vi "ICR_Update_Controls.vi"(7 "Command":T1, 8 "error in (no error)":errorcluster caption="entrée d'erreur (pas d'erreur)", 11 "QMH ICR Cluster":T2) -> (0 "error out":errorcluster caption="sortie d'erreur", 3 "QMH ICR Cluster":T2)   [LabVIEW 2024]
doc: "This VI enables or disables controls according to QMH command."
uses:
  controls/QMH_ICR_Cluster.ctl
  controls/HARDWARE_Resources.ctl
  controls/PROCESSING_Inputs.ctl
  controls/LOOPS_Inputs.ctl
  controls/OPO_Inputs.ctl
  controls/QMH_ICR_Command.ctl
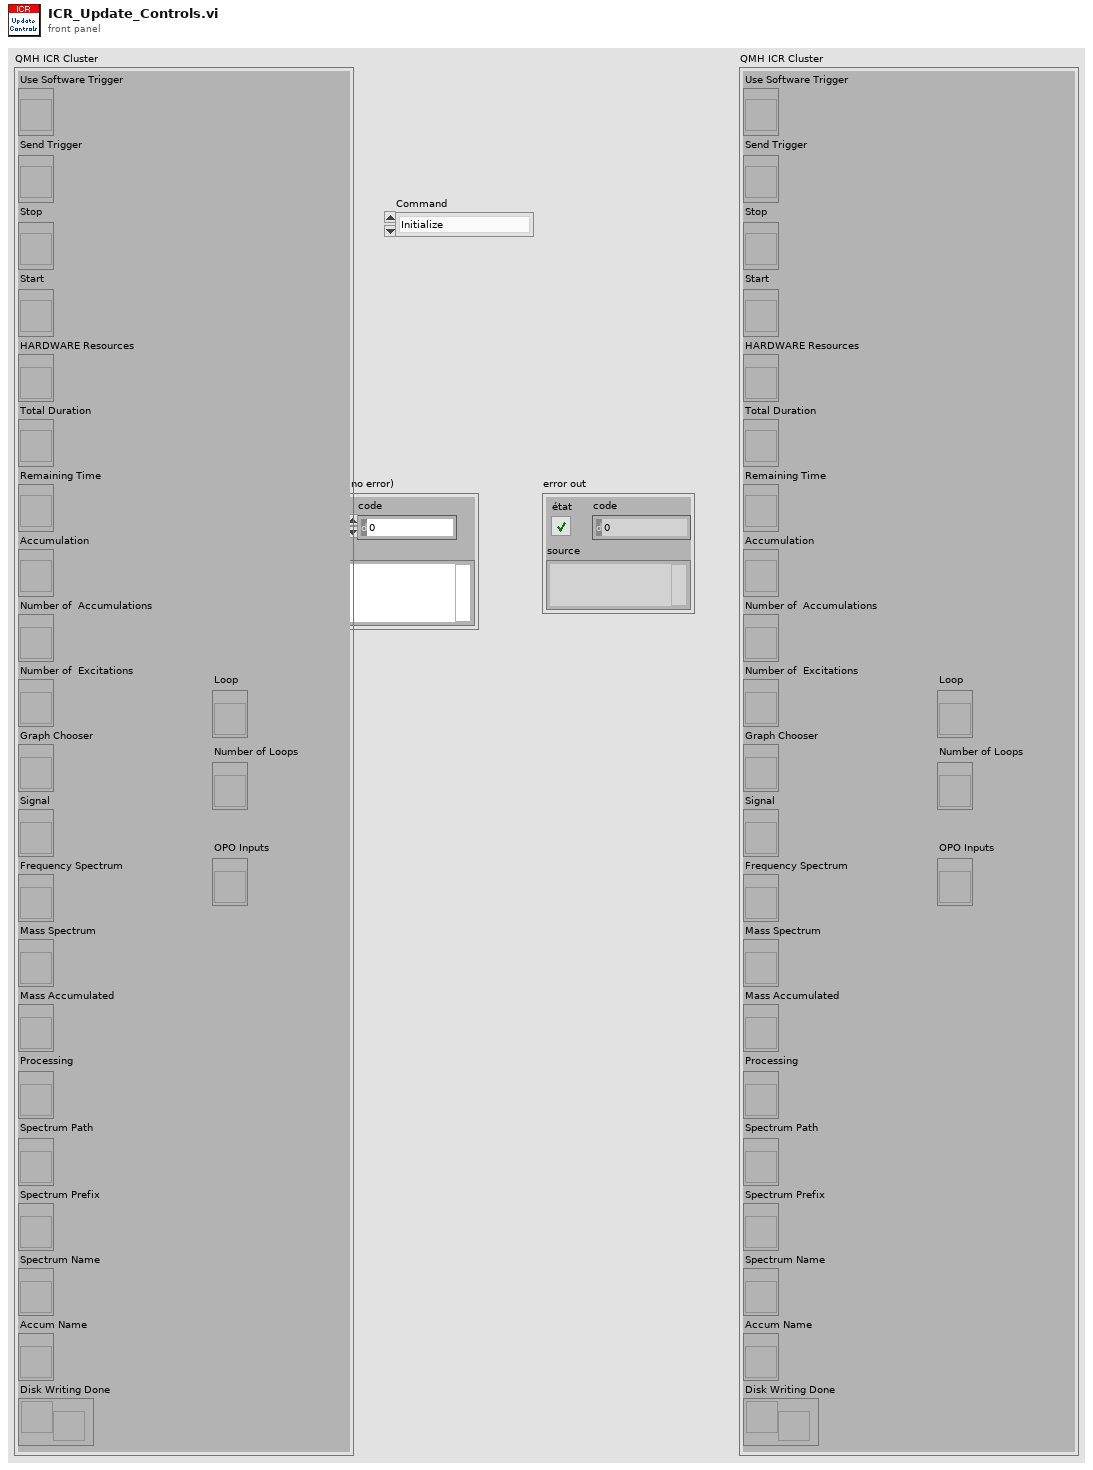
[diagram p1: front panel]
types:
  T1 = typedef "QMH_ICR_Command.ctl" = enum16{"Initialize", "Sequence Loop Setup", "Sequence Setup", "ICR Start", "ICR Stop", "Hardware Setup", "Next Sequence Loop", "Next Accumulation", "Waiting for Trigger", "Sequence Started", "Sequence Finished", "Sequence Loop Done", "Writing Data", "Hardware Reset", "Exit"}
  T2 = typedef "QMH_ICR_Cluster.ctl" = cluster{"Use Software Trigger":refnum<vi>, "Send Trigger":refnum<vi>, "Stop":refnum<vi>, "Start":refnum<vi>, "HARDWARE Resources":refnum<vi>, "Total Duration":refnum<vi>, "Remaining Time":refnum<vi>, "Accumulation":refnum<vi>, "Number of  Accumulations":refnum<vi>, "Number of  Excitations":refnum<vi>, "Graph Chooser":refnum<vi>, "Signal":refnum<vi>, "Frequency Spectrum":refnum<vi>, "Mass Spectrum":refnum<vi>, "Mass Accumulated":refnum<vi>, "Processing":refnum<vi>, "Spectrum Path":refnum<vi>, "Spectrum Prefix":refnum<vi>, "Spectrum Name":refnum<vi>, "Accum Name":refnum<vi>, "Disk Writing Done":refnum<notifier>, "Loop":refnum<vi>, "Number of Loops":refnum<vi>, "OPO Inputs":refnum<vi>}
  T3 = enum32{"Signal", "Frequency Spectrum", "Mass Spectrum", "Mass Accumulated"}
  T4 = enum8{"Enabled", "Disabled", "Disabled and Grayed Out"}
  T5 = typedef "PROCESSING_Inputs.ctl" = cluster{"Reference Mass":dbl, "Cyclotron Freq":dbl, "Magnetron Freq":dbl}
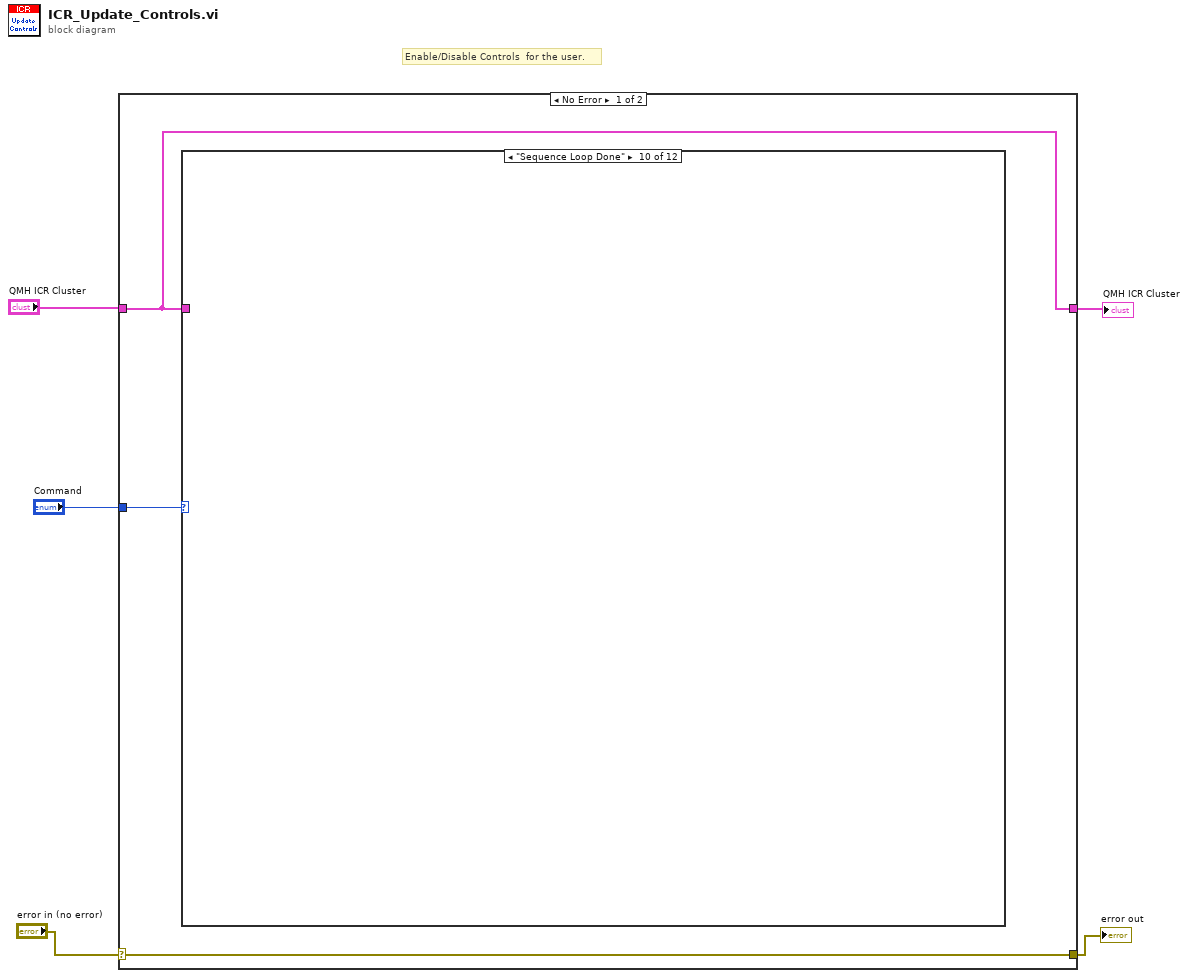
[diagram p0: block diagram]
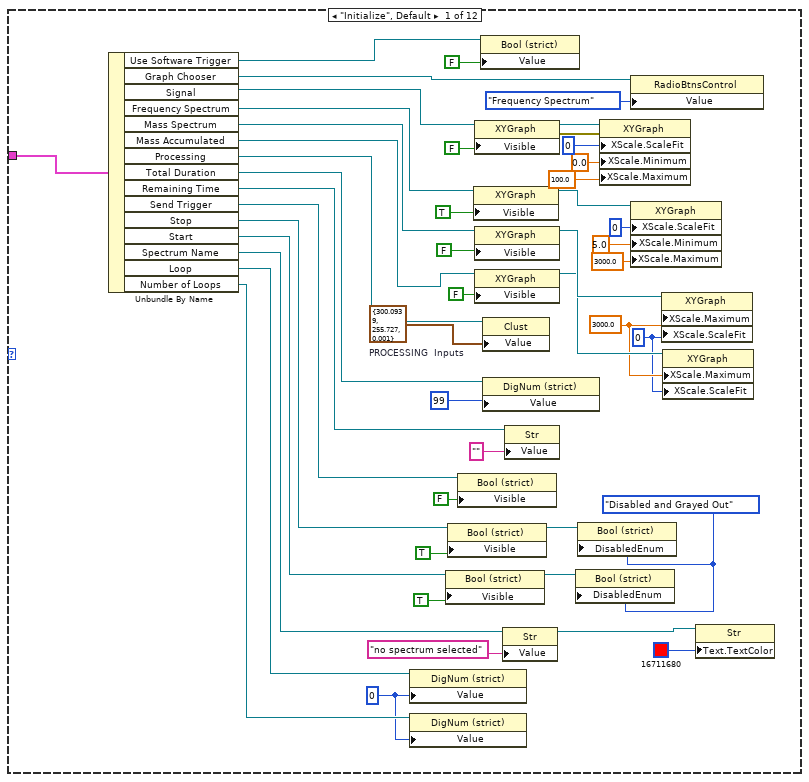
[diagram p2: hidden frame]
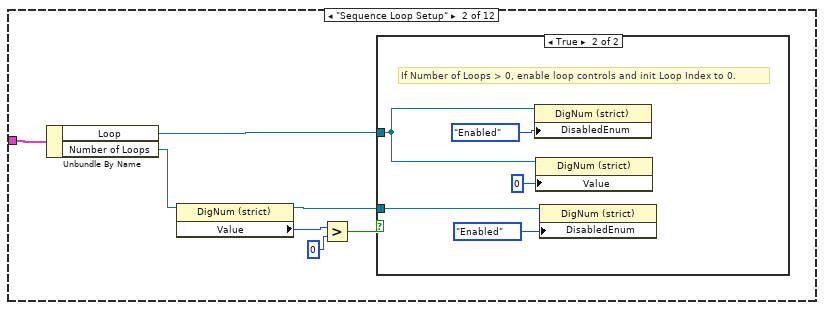
[diagram p3: hidden frame]
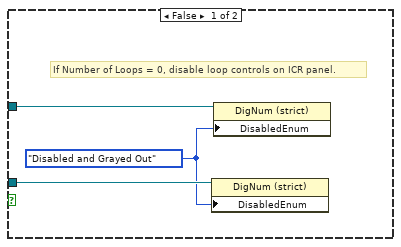
[diagram p4: hidden frame]
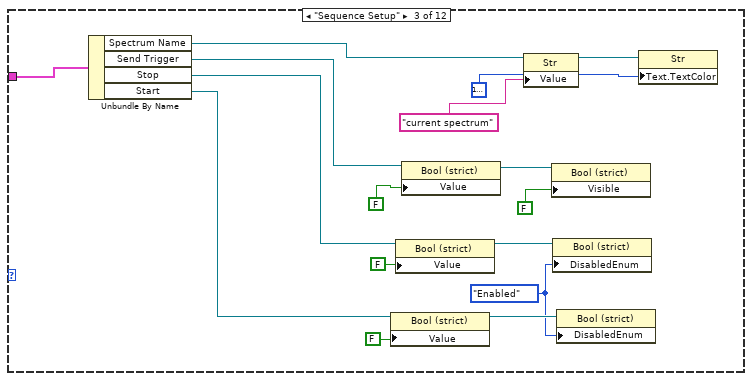
[diagram p5: hidden frame]
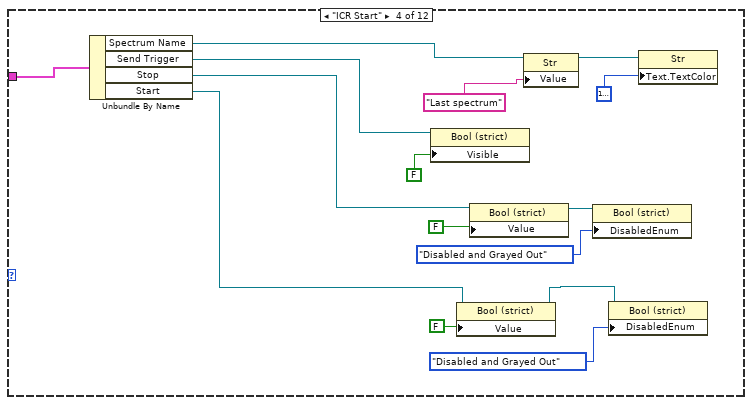
[diagram p6: hidden frame]
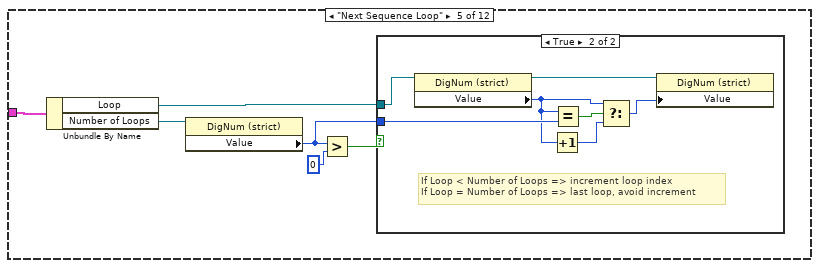
[diagram p7: hidden frame]
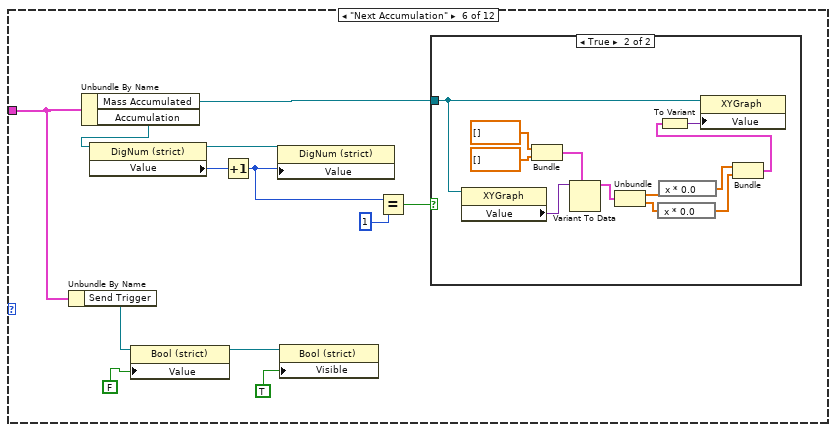
[diagram p9: hidden frame]
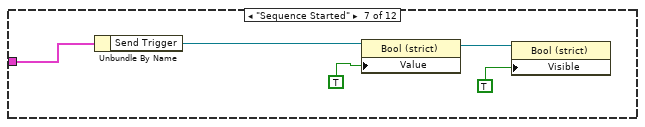
[diagram p11: hidden frame]
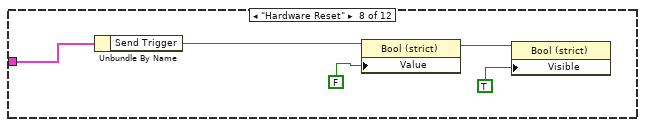
[diagram p12: hidden frame]
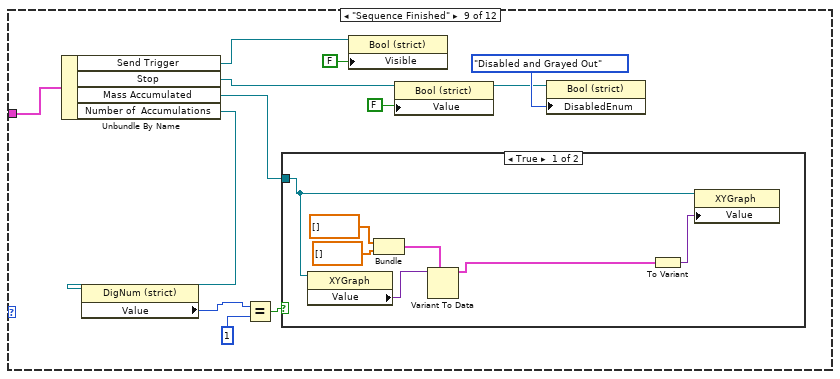
[diagram p13: hidden frame]
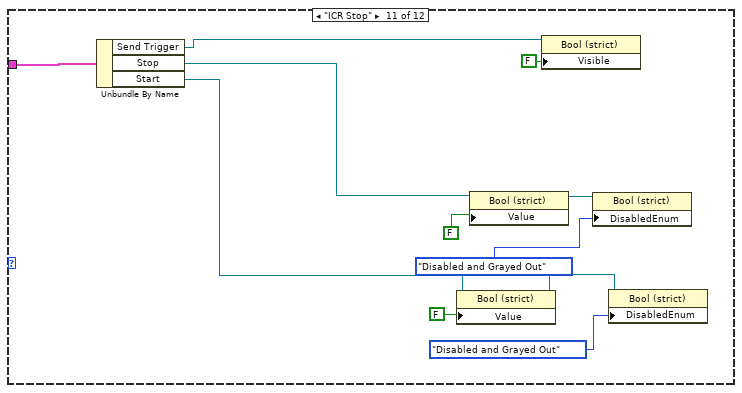
[diagram p15: hidden frame]
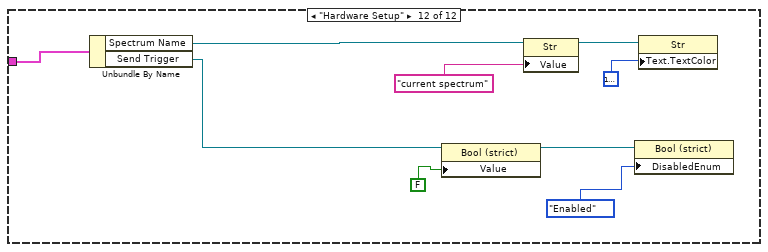
[diagram p16: hidden frame]
diagram:
  # "Enable/Disable Controls  for the user."
  n1 = case shown="No Error" "error in (no error)" {
    selector: "error in (no error)" -> [w8 w190]
    tunnel: "QMH ICR Cluster" -> [w7 w189]
    tunnel: [w8 w190] -> w2
    tunnel: [w7 w189] -> w5
    tunnel: "Command" -> [w6 _]
    frame No Error {
      n2 = case shown="\"Sequence Loop Done\"" w6 {
        tunnel: w7 -> [w32 w63 w87 w102 w108 w117 w144 w149 w161 _ w179 w188]
        frame "Initialize", Default {
          w9 = i16 0 ("Value")
          w16 = u8 0 ("Échelle des X.Ajuster l'échelle")
          w17 = 3000.0 ("Échelle des X.Gamme:Minimum")
          w25 = T4."Disabled and Grayed Out" ("Désactivé")
          w35 = T5 {"Reference Mass"=300.0939, "Cyclotron Freq"=255.727, "Magnetron Freq"=0.001}  # PROCESSING  Inputs
          n3 = Unbundle By Name(w32) -> ("Use Software Trigger"=w48:refnum<vi>, "Graph Chooser"=w49:refnum<vi>, "Signal"=w50:refnum<vi>, "Frequency Spectrum"=w51:refnum<vi>, "Mass Spectrum"=w52:refnum<vi>, "Mass Accumulated"=w36:refnum<vi>, "Processing"=w42:refnum<vi>, "Total Duration"=w46:refnum<vi>, "Remaining Time"=w44:refnum<vi>, "Send Trigger"=w29:refnum<vi>, "Stop"=w39:refnum<vi>, "Start"=w26:refnum<vi>, "Spectrum Name"=w30:refnum<vi>, "Loop"=w11:refnum<vi>, "Number of Loops"=w10:refnum<vi>)
          n4 = property class="DigNum (strict)"(reference=w11, "Value"=w9) -> ()  [unwired: 1 in, 2 out]
          n5 = property class="DigNum (strict)"(reference=w10, "Value"=w9) -> ()  [unwired: 1 in, 2 out]
          n6 = property class="Bool (strict)"(reference=w26, "Visible"=TRUE) -> (reference out=w28:refnum<vi>)  [unwired: 1 in, 1 out]
          n7 = property class="Bool (strict)"(reference=w39, "Visible"=TRUE) -> (reference out=w34:refnum<vi>)  [unwired: 1 in, 1 out]
          n8 = property class="Bool (strict)"(reference=w29, "Visible"=FALSE) -> ()  [unwired: 1 in, 2 out]
          n9 = property class="XYGraph"(reference=w51, "Visible"=TRUE) -> (reference out=w21:refnum<vi>)  [unwired: 1 in, 1 out]
          n10 = property class="XYGraph"(reference=w50, "Visible"=FALSE) -> (reference out=w24:refnum<vi>, error out=w23:errorcluster)  [unwired: 1 in]
          n11 = property class="XYGraph"(reference=w52, "Visible"=FALSE) -> (reference out=w19:refnum<vi>)  [unwired: 1 in, 1 out]
          n12 = property class="XYGraph"(reference=w36, "Visible"=FALSE) -> (reference out=w18:refnum<vi>)  [unwired: 1 in, 1 out]
          n13 = property class="Bool (strict)"(reference=w48, "Value"=FALSE ("Valeur")) -> ()  [unwired: 1 in, 2 out]
          n14 = property class="Clust"(reference=w42, "Value"=w35) -> ()  [unwired: 1 in, 2 out]
          n15 = property class="DigNum (strict)"(reference=w46, "Value"=99) -> ()  [unwired: 1 in, 2 out]
          n16 = property class="Str"(reference=w30, "Value"="no spectrum selected" ("Valeur")) -> (reference out=w40:refnum<vi>)  [unwired: 1 in, 1 out]
          n17 = property class="Str"(reference=w44, "Value"="" ("Valeur")) -> ()  [unwired: 1 in, 2 out]
          n18 = property class="Bool (strict)"(reference=w28, "DisabledEnum"=w25) -> ()  [unwired: 1 in, 2 out]
          n19 = property class="Bool (strict)"(reference=w34, "DisabledEnum"=w25) -> ()  [unwired: 1 in, 2 out]
          n20 = property class="XYGraph"(reference=w24, error in=w23, "XScale.ScaleFit"=u8 0 ("Échelle des X.Ajuster l'échelle"), "XScale.Minimum"=0.0 ("Échelle des X.Gamme:Minimum"), "XScale.Maximum"=100.0 ("Échelle des X.Gamme:Maximum")) -> ()  [unwired: 2 out]
          n21 = property class="RadioBtnsControl"(reference=w49, "Value"=T3."Frequency Spectrum" ("Graph Chooser")) -> ()  [unwired: 1 in, 2 out]
          n22 = property class="XYGraph"(reference=w21, "XScale.ScaleFit"=u8 0 ("Échelle des X.Ajuster l'échelle"), "XScale.Minimum"=5.0 ("Échelle des X.Gamme:Minimum"), "XScale.Maximum"=3000.0 ("Échelle des X.Gamme:Maximum")) -> ()  [unwired: 1 in, 2 out]
          n23 = property class="XYGraph"(reference=w19, "XScale.Maximum"=w17, "XScale.ScaleFit"=w16) -> ()  [unwired: 1 in, 2 out]
          n24 = property class="XYGraph"(reference=w18, "XScale.Maximum"=w17, "XScale.ScaleFit"=w16) -> ()  [unwired: 1 in, 2 out]
          n25 = property on="Nœud de propriété" class="Str"(reference=w40, "Text.TextColor"=u32 16711680) -> ()  [unwired: 1 in, 2 out]
        }
        frame "Sequence Loop Setup" {
          n26 = Unbundle By Name(w63) -> ("Loop"=w60:refnum<vi>, "Number of Loops"=w58:refnum<vi>)
          n27 = property class="DigNum (strict)"(reference=w58) -> (reference out=w57:refnum<vi>, "Value"=w59:i16)  [unwired: 1 in, 1 out]
          n28 = Greater?(x=w59, y=i16 0) -> (0:w62:bool)
          n29 = case shown="True" w62 {
            tunnel: w60 -> [w66 w69]
            tunnel: w57 -> [w65 w71]
            frame False {
              w64 = T4."Disabled and Grayed Out" ("Disabled")
              # "If Number of Loops = 0, disable loop controls on ICR panel."
              n30 = property class="DigNum (strict)"(reference=w65, "DisabledEnum"=w64) -> ()  [unwired: 1 in, 2 out]
              n31 = property class="DigNum (strict)"(reference=w66, "DisabledEnum"=w64) -> ()  [unwired: 1 in, 2 out]
            }
            frame True {
              # "If Number of Loops > 0, enable loop controls and init Loop Index to 0."
              n32 = property class="DigNum (strict)"(reference=w69, "DisabledEnum"=T4."Enabled" ("Disabled")) -> ()  [unwired: 1 in, 2 out]
              n33 = property class="DigNum (strict)"(reference=w69, "Value"=i16 0) -> ()  [unwired: 1 in, 2 out]
              n34 = property class="DigNum (strict)"(reference=w71, "DisabledEnum"=T4."Enabled" ("Disabled")) -> ()  [unwired: 1 in, 2 out]
            }
          }
        }
        frame "Sequence Setup" {
          w72 = T4."Enabled" ("Désactivé")
          n35 = Unbundle By Name(w87) -> ("Spectrum Name"=w85:refnum<vi>, "Send Trigger"=w82:refnum<vi>, "Stop"=w77:refnum<vi>, "Start"=w73:refnum<vi>)
          n36 = property class="Bool (strict)"(reference=w73, "Value"=FALSE ("Valeur")) -> (reference out=w75:refnum<vi>)  [unwired: 1 in, 1 out]
          n37 = property class="Bool (strict)"(reference=w77, "Value"=FALSE ("Valeur")) -> (reference out=w78:refnum<vi>)  [unwired: 1 in, 1 out]
          n38 = property class="Bool (strict)"(reference=w82, "Value"=FALSE ("Valeur")) -> (reference out=w81:refnum<vi>)  [unwired: 1 in, 1 out]
          n39 = property class="Str"(reference=w85, "Value"="current spectrum" ("Valeur")) -> (reference out=w83:refnum<vi>)  [unwired: 1 in, 1 out]
          n40 = property class="Bool (strict)"(reference=w81, "Visible"=FALSE) -> ()  [unwired: 1 in, 2 out]
          n41 = property class="Bool (strict)"(reference=w78, "DisabledEnum"=w72) -> ()  [unwired: 1 in, 2 out]
          n42 = property class="Bool (strict)"(reference=w75, "DisabledEnum"=w72) -> ()  [unwired: 1 in, 2 out]
          n43 = property on="Nœud de propriété" class="Str"(reference=w83, "Text.TextColor"=u32 16777222) -> ()  [unwired: 1 in, 2 out]
        }
        frame "ICR Start" {
          n44 = Unbundle By Name(w102) -> ("Spectrum Name"=w101:refnum<vi>, "Send Trigger"=w89:refnum<vi>, "Stop"=w97:refnum<vi>, "Start"=w94:refnum<vi>)
          n45 = property class="Bool (strict)"(reference=w89, "Visible"=FALSE) -> ()  [unwired: 1 in, 2 out]
          n46 = property class="Bool (strict)"(reference=w94, "Value"=FALSE ("Valeur")) -> (reference out=w95:refnum<vi>)  [unwired: 1 in, 1 out]
          n47 = property class="Bool (strict)"(reference=w97, "Value"=FALSE ("Valeur")) -> (reference out=w98:refnum<vi>)  [unwired: 1 in, 1 out]
          n48 = property class="Str"(reference=w101, "Value"="Last spectrum" ("Valeur")) -> (reference out=w99:refnum<vi>)  [unwired: 1 in, 1 out]
          n49 = property class="Bool (strict)"(reference=w98, "DisabledEnum"=T4."Disabled and Grayed Out" ("Désactivé")) -> ()  [unwired: 1 in, 2 out]
          n50 = property class="Bool (strict)"(reference=w95, "DisabledEnum"=T4."Disabled and Grayed Out" ("Désactivé")) -> ()  [unwired: 1 in, 2 out]
          n51 = property on="Nœud de propriété" class="Str"(reference=w99, "Text.TextColor"=u32 16777222) -> ()  [unwired: 1 in, 2 out]
        }
        frame "Next Sequence Loop" {
          n52 = Unbundle By Name(w108) -> ("Loop"=w104:refnum<vi>, "Number of Loops"=w106:refnum<vi>)
          n53 = property class="DigNum (strict)"(reference=w106) -> ("Value"=w103:i16)  [unwired: 1 in, 2 out]
          n54 = Greater?(x=w103, y=i16 0) -> (0:w107:bool)
          n55 = case shown="True" w107 {
            tunnel: w104 -> [_ w115]
            tunnel: w103 -> [_ w114]
            frame False {
            }
            frame True {
              # "If Loop < Number of Loops => increment loop index\nIf Loop = Number of Loops => last loop, avoid increment"
              n56 = property class="DigNum (strict)"(reference=w115) -> (reference out=w112:refnum<vi>, "Value"=w111:i16)  [unwired: 1 in, 1 out]
              n57 = Increment(x=w111) -> (x+1=w110:i16)
              n58 = Equal?(x=w111, y=w114) -> (x = y?=w113:bool)
              n59 = Select(t=w111, s=w113, f=w110) -> (s? t:f=w109:i16)
              n60 = property class="DigNum (strict)"(reference=w112, "Value"=w109) -> ()  [unwired: 1 in, 2 out]
            }
          }
        }
        frame "Next Accumulation" {
          n61 = Unbundle By Name(w117) -> ("Send Trigger"=w116:refnum<vi>)
          n62 = Unbundle By Name(w117) -> ("Mass Accumulated"=w127:refnum<vi>, "Accumulation"=w122:refnum<vi>)
          n63 = property class="DigNum (strict)"(reference=w122) -> (reference out=w124:refnum<vi>, "Value"=w123:i16)  [unwired: 1 in, 1 out]
          n64 = property class="Bool (strict)"(reference=w116, "Value"=FALSE ("Valeur")) -> (reference out=w120:refnum<vi>)  [unwired: 1 in, 1 out]
          n65 = Increment(x=w123) -> (x+1=w121:i16)
          n66 = property class="DigNum (strict)"(reference=w124, "Value"=w121) -> ()  [unwired: 1 in, 2 out]
          n67 = property class="Bool (strict)"(reference=w120, "Visible"=TRUE) -> ()  [unwired: 1 in, 2 out]
          n68 = Equal?(x=w121, y=i16 1) -> (x = y?=w126:bool)
          n69 = case shown="True" w126 {
            tunnel: w127 -> [_ w128]
            frame False {
            }
            frame True {
              n70 = property class="XYGraph"(reference=w128) -> ("Value"=w138:variant)  [unwired: 1 in, 2 out]
              n71 = Bundle("Tableau 2"=dbl[] [], "Tableau 2"=dbl[] []) -> (w135:cluster{"Tableau 2":dbl[], "Tableau 2":dbl[]})  [unwired: 1 in]
              n72 = Variant To Data(type=w135, Variant=w138) -> (data=w134:cluster{"Tableau 2":dbl[], "Tableau 2":dbl[]})  [unwired: 1 in, 1 out]
              n73 = Unbundle(w134) -> ("Tableau 2"=w131:dbl[], "Tableau 2"=w130:dbl[])
              n74 = expression code="x * 0.0"(w130) -> (w133:dbl[])
              n75 = expression code="x * 0.0"(w131) -> (w129:dbl[])
              n76 = Bundle("Tableau 2"=w129, "Tableau 2"=w133) -> (w132:cluster{"Tableau 2":dbl[], "Tableau 2":dbl[]})  [unwired: 1 in]
              n77 = To Variant(anything=w132) -> (Variant=w136:variant)
              n78 = property class="XYGraph"(reference=w128, "Value"=w136) -> ()  [unwired: 1 in, 2 out]
            }
          }
        }
        frame "Sequence Started" {
          n79 = Unbundle By Name(w144) -> ("Send Trigger"=w143:refnum<vi>)
          n80 = property class="Bool (strict)"(reference=w143, "Value"=TRUE ("Valeur")) -> (reference out=w142:refnum<vi>)  [unwired: 1 in, 1 out]
          n81 = property class="Bool (strict)"(reference=w142, "Visible"=TRUE) -> ()  [unwired: 1 in, 2 out]
        }
        frame "Hardware Reset" {
          n82 = Unbundle By Name(w149) -> ("Send Trigger"=w148:refnum<vi>)
          n83 = property class="Bool (strict)"(reference=w148, "Value"=FALSE ("Valeur")) -> (reference out=w147:refnum<vi>)  [unwired: 1 in, 1 out]
          n84 = property class="Bool (strict)"(reference=w147, "Visible"=TRUE) -> ()  [unwired: 1 in, 2 out]
        }
        frame "Sequence Finished" {
          n85 = Unbundle By Name(w161) -> ("Send Trigger"=w151:refnum<vi>, "Stop"=w152:refnum<vi>, "Mass Accumulated"=w159:refnum<vi>, "Number of  Accumulations"=w160:refnum<vi>)
          n86 = property class="DigNum (strict)"(reference=w160) -> ("Value"=w156:i16)  [unwired: 1 in, 2 out]
          n87 = Equal?(x=w156, y=i16 1) -> (x = y?=w157:bool)
          n88 = case shown="True" w157 {
            tunnel: w159 -> [w162 _]
            frame True {
              n89 = property class="XYGraph"(reference=w162) -> ("Value"=w166:variant)  [unwired: 1 in, 2 out]
              n90 = Bundle("Tableau"=dbl[] [], "Tableau 2"=dbl[] []) -> (w165:cluster{"Tableau":dbl[], "Tableau 2":dbl[]})  [unwired: 1 in]
              n91 = Variant To Data(type=w165, Variant=w166) -> (data=w163:cluster{"Tableau":dbl[], "Tableau 2":dbl[]})  [unwired: 1 in, 1 out]
              n92 = To Variant(anything=w163) -> (Variant=w164:variant)
              n93 = property class="XYGraph"(reference=w162, "Value"=w164) -> ()  [unwired: 1 in, 2 out]
            }
            frame False {
            }
          }
          n94 = property class="Bool (strict)"(reference=w151, "Visible"=FALSE) -> ()  [unwired: 1 in, 2 out]
          n95 = property class="Bool (strict)"(reference=w152, "Value"=FALSE ("Valeur")) -> (reference out=w154:refnum<vi>)  [unwired: 1 in, 1 out]
          n96 = property class="Bool (strict)"(reference=w154, "DisabledEnum"=T4."Disabled and Grayed Out" ("Désactivé")) -> ()  [unwired: 1 in, 2 out]
        }
        frame "Sequence Loop Done" {
        }
        frame "ICR Stop" {
          n97 = Unbundle By Name(w179) -> ("Send Trigger"=w169:refnum<vi>, "Stop"=w176:refnum<vi>, "Start"=w173:refnum<vi>)
          n98 = property class="Bool (strict)"(reference=w173, "Value"=FALSE ("Valeur")) -> (reference out=w174:refnum<vi>)  [unwired: 1 in, 1 out]
          n99 = property class="Bool (strict)"(reference=w176, "Value"=FALSE ("Valeur")) -> (reference out=w178:refnum<vi>)  [unwired: 1 in, 1 out]
          n100 = property class="Bool (strict)"(reference=w169, "Visible"=FALSE) -> ()  [unwired: 1 in, 2 out]
          n101 = property class="Bool (strict)"(reference=w178, "DisabledEnum"=T4."Disabled and Grayed Out" ("Désactivé")) -> ()  [unwired: 1 in, 2 out]
          n102 = property class="Bool (strict)"(reference=w174, "DisabledEnum"=T4."Disabled and Grayed Out" ("Désactivé")) -> ()  [unwired: 1 in, 2 out]
        }
        frame "Hardware Setup" {
          n103 = Unbundle By Name(w188) -> ("Spectrum Name"=w186:refnum<vi>, "Send Trigger"=w182:refnum<vi>)
          n104 = property class="Bool (strict)"(reference=w182, "Value"=FALSE ("Valeur")) -> (reference out=w181:refnum<vi>)  [unwired: 1 in, 1 out]
          n105 = property class="Str"(reference=w186, "Value"="current spectrum" ("Valeur")) -> (reference out=w184:refnum<vi>)  [unwired: 1 in, 1 out]
          n106 = property class="Bool (strict)"(reference=w181, "DisabledEnum"=T4."Enabled" ("Désactivé")) -> ()  [unwired: 1 in, 2 out]
          n107 = property on="Nœud de propriété" class="Str"(reference=w184, "Text.TextColor"=u32 16777222) -> ()  [unwired: 1 in, 2 out]
        }
      }
    }
    frame Error {
    }
  }
  "error out" <- w2
  "QMH ICR Cluster" <- w5
